vi "FPGA_SICK Check for overflows.vi"(1 "EN mask overflow bytes":bool, 2 "Data chunk in":u16, 3 "En overflow replacement":bool) -> (0 "Data chunk out":u16)   [LabVIEW 2009]
uses:
  <vilib>/rvi/DataTransferAndStorage/Container/XNode/niFpgaContainer.xnode
  <vilib>/rvi/Memory/Memory_Emulation/nirvimemoryEmulationManagerCache_GetValue.vi
  <vilib>/rvi/Memory/Memory_Emulation/nirvimemoryEmulationManagerCache_InsertValue.vi
  <vilib>/rvi/DataTransferAndStorage/Container/Common/niFpgaContainerGetUniqueNameForEmu.vi
  <vilib>/Utility/error.llb/Clear Errors.vi
  <vilib>/rvi/Memory/Memory_Emulation/nirvimemoryEmulationManagerCache_SetValue.vi
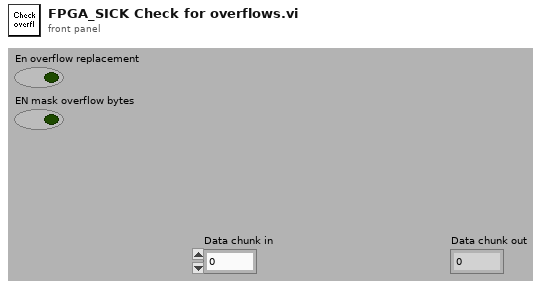
[diagram p1: front panel]
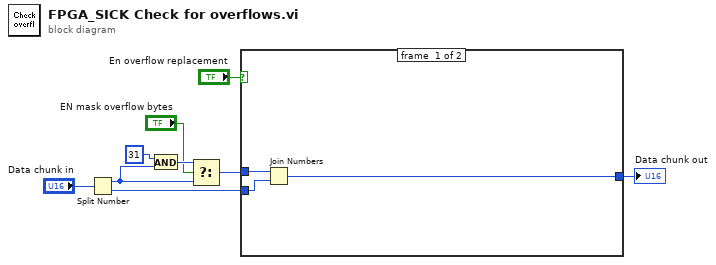
[diagram p0: block diagram]
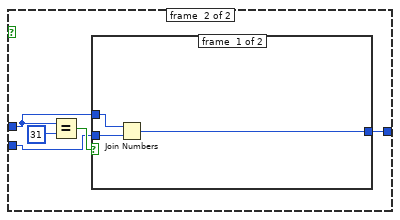
[diagram p2: hidden frame]
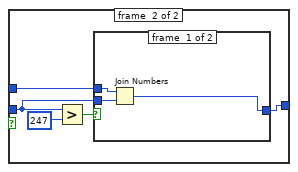
[diagram p3: hidden frame]
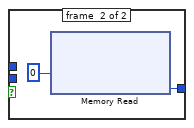
[diagram p4: hidden frame]
diagram:
  n1 = Split Number(x="Data chunk in") -> (hi(x)=w2:u8, lo(x)=w6:u8)
  n2 = And(x=u8 31, y=w2) -> (x .and. y?=w3:u8)
  n3 = Select(t=w3, s="EN mask overflow bytes", f=w2) -> (s? t:f=w4:u8)
  n4 = case shown="False" "En overflow replacement" {
    tunnel: [w10 w16] -> w8
    tunnel: w4 -> [w12 w14]
    tunnel: w6 -> [w11 w13]
    frame #0 {
      n5 = Join Numbers(hi=w12, lo=w11) -> ((hi.lo)=w10:u16)
    }
    frame #1 {
      n6 = Equal?(x=w14, y=u8 31) -> (x = y?=w15:bool)
      n7 = case shown="True" w15 {
        tunnel: [w19 w23] -> w16
        tunnel: w13 -> [w20 w21]
        tunnel: w14 -> [w18 w22]
        frame #0 {
          n8 = Join Numbers(hi=w18, lo=w20) -> ((hi.lo)=w19:u16)
        }
        frame #1 {
          n9 = Greater?(x=w21, y=u8 247) -> (0:w24:bool)
          n10 = case shown="True" w24 {
            tunnel: [w26 w29] -> w23
            tunnel: w21 -> [w28 _]
            tunnel: w22 -> [w27 _]
            frame #0 {
              n11 = Join Numbers(hi=w27, lo=w28) -> ((hi.lo)=w26:u16)
            }
            frame #1 {
              n12 = xnode ("Memory Read")("Address"=u32 0) -> ("Data"=w29:u16)  [unwired: 1 in, 1 out]
            }
          }
        }
      }
    }
  }
  "Data chunk out" <- w8
